vi "Multi.vi"(8 "error in (no error)":errorcluster, 10 "Data Sources":refnum<class "Aux Data Source.lvclass">[](array[class]), 11 "Multi in":refnum<class "Multi.lvclass">) -> (0 "error out":errorcluster, 3 "Multi out":refnum<class "Multi.lvclass">)   [LabVIEW 2023, in "Multi.lvclass"]
uses:
  Multi.lvclass
  Aux Data Source/Aux Data Source.lvclass
  Multi.lvclass/Multi.ctl
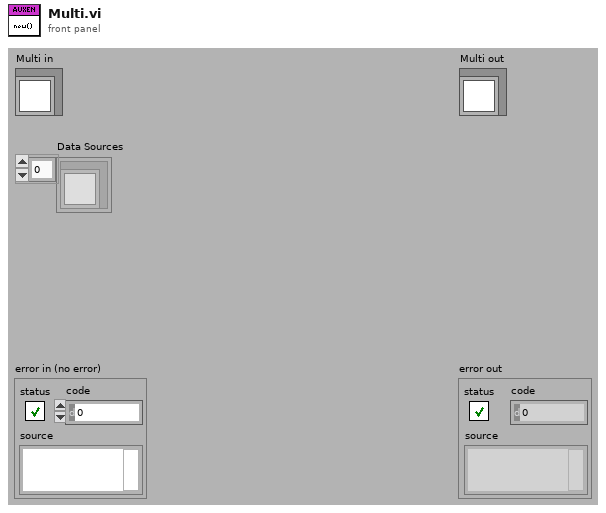
[diagram p1: front panel]
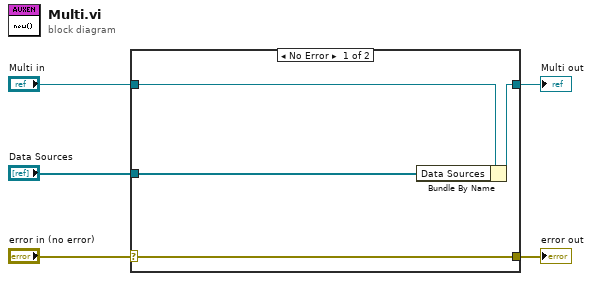
[diagram p0: block diagram]
diagram:
  n1 = case shown="No Error" "error in (no error)" {
    selector: "error in (no error)" -> [w9 w10]
    tunnel: [w9 w10] -> w4
    tunnel: [w7 w11] -> w2
    tunnel: "Multi in" -> [w8 w11]
    tunnel: "Data Sources" -> [w6 _]
    frame No Error {
      n2 = Bundle By Name(cluster=w8, "Data Sources"=w6) -> (w7:refnum<class "Multi.lvclass">)
    }
    frame Error {
    }
  }
  "error out" <- w4
  "Multi out" <- w2
